vi "basic - BITE Transfer Test.vi"() -> ()   [LabVIEW 2020]
uses:
  _polimorphicInstances/session/Fdx Create Session (Generic-Board).vi
  _polimorphicInstances/session/Fdx Close Session (Board).vi
  AIM664LV.lvlib
panel:
  out "Error Message":string
  out "error out":errorcluster
  in  "SrvName":string="local"
  in  "Board ID":u32
  # "ARINC 664 BITE Transfer Test"
  # "Overview: Performs some transfer tests using available port resources of one FDX board. This function will determine the number of ports on the board. If only two ports, it will test them against each other. If four ports are used, Port 1 and Port 2 will be tested against each other and Port 3 and Port 4 will be tested against each other. \nPort 1 and Port 2 must be connected with a Loop-Back cable (crossover), if available Port 3 and Port 4 must be connected with a Loop-Back cable (crossover).\nThe resources of the board under test shall be not logged in.\n\nRequirement: One AIM ARINC-664 board with installed AIM ARINC 664 BSP.\nRestrictions: None.\nInstruction:\n1. Select the Board ID (0 if you have only one board in your system).\n2. Run the VI.\n3. If no error is presented, the test was performed correctly."
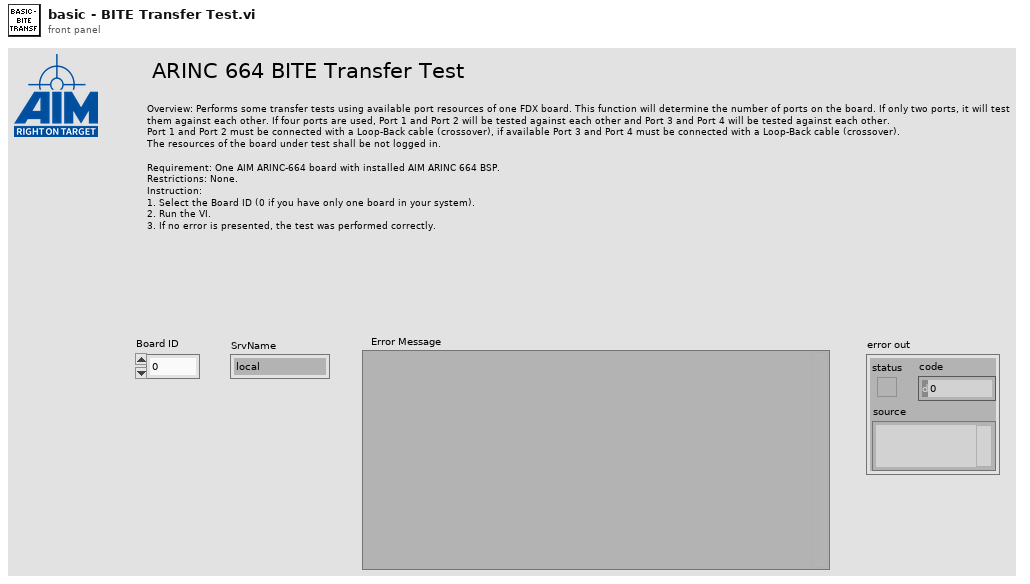
[diagram p1: front panel]
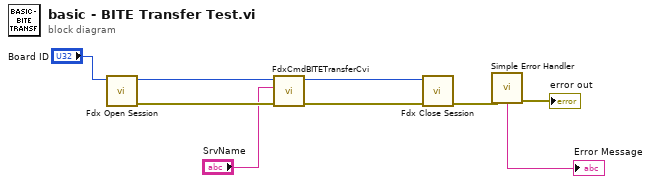
[diagram p0: block diagram]
diagram:
  n1 = call-poly "Fdx Open Session.vi"("board"="Board ID") -> ("error out"=w9:errorcluster, "InstrumentHandle_board out"=w2:u32)  [unwired: 8 in, 1 out]
  n2 = call "FdxCmdBITETransferCvi.vi"("error in"=w9, "SrvName"="SrvName", "Board_ResourceID"=w2) -> ("error out"=w8:errorcluster, "Board_ResourceID Out"=w1:u32)  [unwired: 7 in]
  n3 = call-poly "Fdx Close Session.vi"("error in (no error)"=w8, "InstrumentHandle_board in"=w1) -> ("error out"=w7:errorcluster)  [unwired: 9 in]
  n4 = call <vilib>:"Simple Error Handler.vi"("error in (no error)"=w7) -> ("error out"=→"error out":errorcluster, "message"=→"Error Message":string)  [unwired: 4 in, 3 out]
